vi "TestCloneAPI.vi"() -> ()   [LabVIEW 2014, in "AnalysisModule.lvlib"]
uses:
  AnalysisModule.lvlib
  TestInfo.ctl
  <userlib>/NIST/ModuleAdminLib/CloneRegistration/CloneRegistration.lvclass
  <userlib>/NIST/ModuleAdminLib/ModuleAdmin/ModuleAdmin.lvclass/ModuleAdmin.ctl
  <userlib>/NIST/ModuleAdminLib/ModuleAdmin/ModuleAdmin.lvclass
  PublicAPI/Arguments/Broadcasts/clDidInit.ctl
  PublicAPI/Arguments/Requests/clStopArgument.ctl
  <userlib>/NIST/ModuleAdminLib/ModuleAdmin/Accessors/Read CloneRegRef.vi
  <userlib>/NIST/ModuleAdminLib/ModuleAdmin/Accessors/Write CloneRegRef.vi
  AnalysisPlugins/AnalysisPluginBaseClass/AnalysisPluginsBase.lvclass
panel:
  in  "btnPref":bool
  out "error out":errorcluster
  in  "TimeStamp":dbl format="%.6f"
  in  "btnLoadPlugin":bool
  in  "SampleDataArray":cluster{"dSampleData":dbl[], "iActualPts":i32}[](array[cluster])=[{"dSampleData"=array[4800 elements], "iActualPts"=4800}, {"dSampleData"=array[4800 elements], "iActualPts"=4800}, {"dSampleData"=array[4800 elements], "iActualPts"=4800}, {"dSampleData"=array[4800 elements], "iActualPts"=4800}, {"dSampleData"=array[4800 elements], "iActualPts"=4800}, {"dSampleData"=array[4800 elements], "iActualPts"=4800}, {"dSampleData"=array[4800 elements], "iActualPts"=4800}, {"dSampleData"=array[4800 elements], "iActualPts"=4800}]
  in  "Show Panel":bool=TRUE
  in  "Plugin Type":u16(ring) items=["None", "PMU"]
  in  "btnWriteSamples":bool
  out "Path":path
  in  "btnRequestINIPath":bool
  in  "btnRemove":bool
  out "Status Log":string
  out "Active Modules (Array)":string[](array[string])
  in  "btnAdd":bool
  in  "btnStop":bool
  in  "Select Module":i32(ring)=-1 caption="Select Module to send Request" items=["All"=-1, "4140005"=4140005]
  # "Hidden"
  # "Visible"
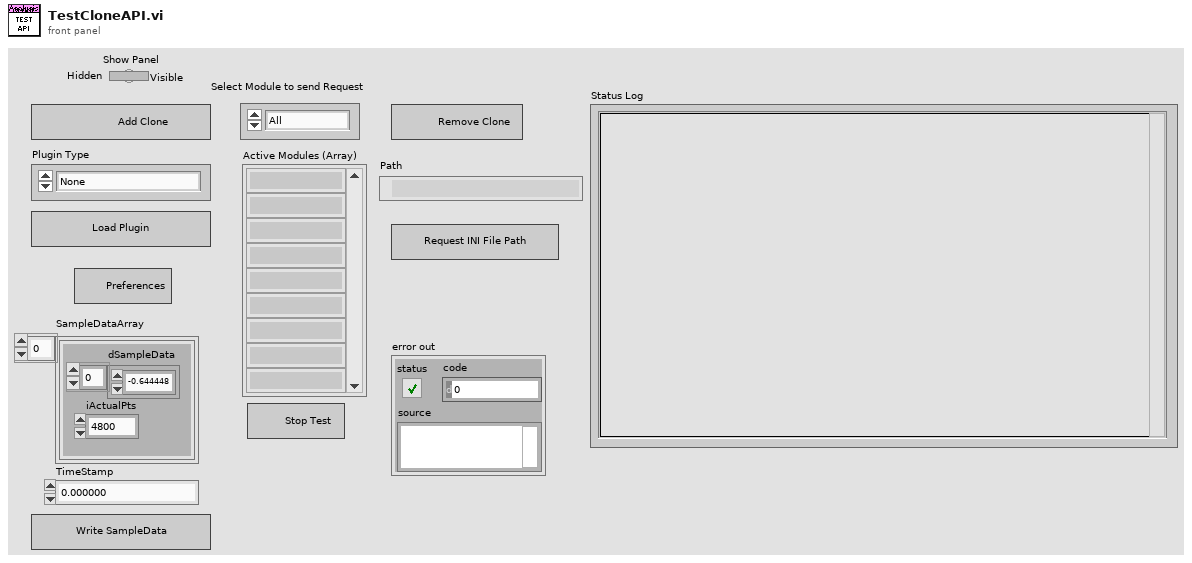
[diagram p1: front panel]
types:
  T1 = typedef "AnalysisModule.lvlib/TestInfo.ctl" = cluster{"PluginIniFilePaths":path[]}
  T2 = typedef "AnalysisModule.lvlib/clBroadcastEvents.ctl" = cluster{"DidInit":refnum<user-event>, "StatusUpdate":refnum<user-event>, "ErrorReport":refnum<user-event>, "DidStop":refnum<user-event>, "PathToINI":refnum<user-event>, "Config":refnum<user-event>, "ResultReport":refnum<user-event>}
  T3 = typedef "AnalysisModule.lvlib/clDidInit.ctl" = cluster{"Init?":bool, "ModuleAdmin":refnum<class "ModuleAdmin.lvclass">}
  T4 = typedef "AnalysisModule.lvlib/clStopArgument.ctl" = cluster{"Exit via Stop Module Req?":bool, "Wait for Module to stop?":bool, "ModuleAdmin":refnum<class "ModuleAdmin.lvclass">}
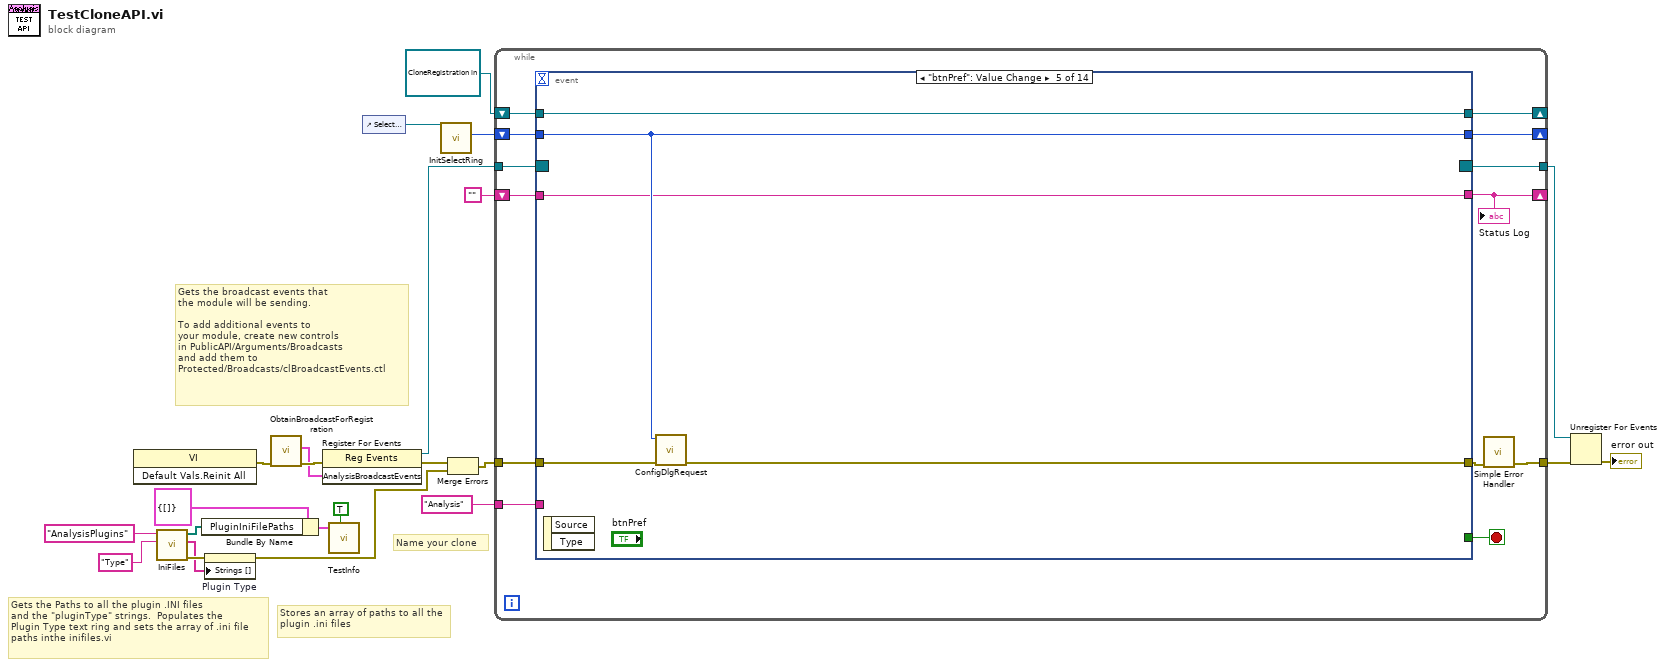
[diagram p0: block diagram]
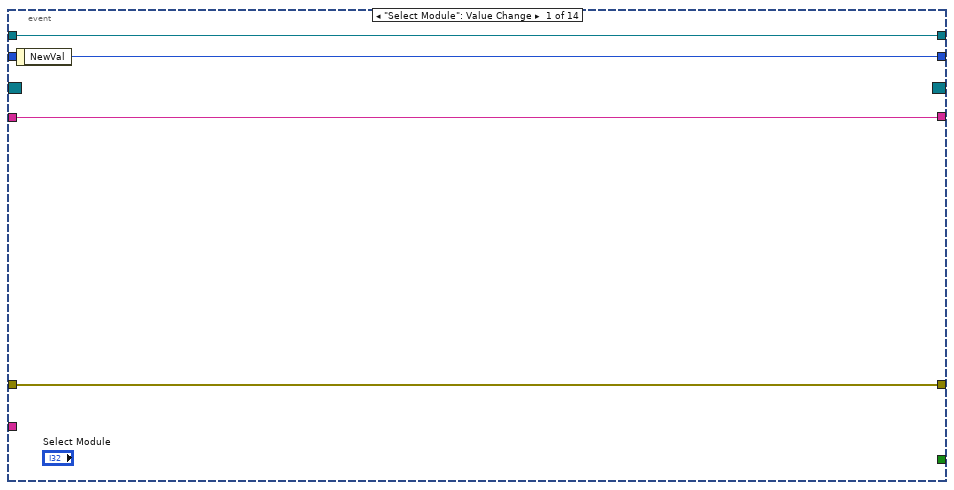
[diagram p2: hidden frame]
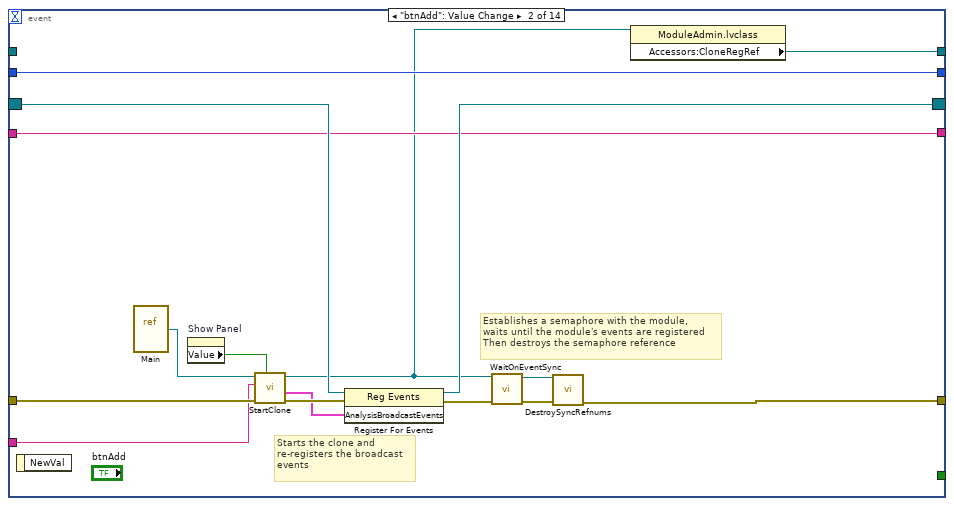
[diagram p3: hidden frame]
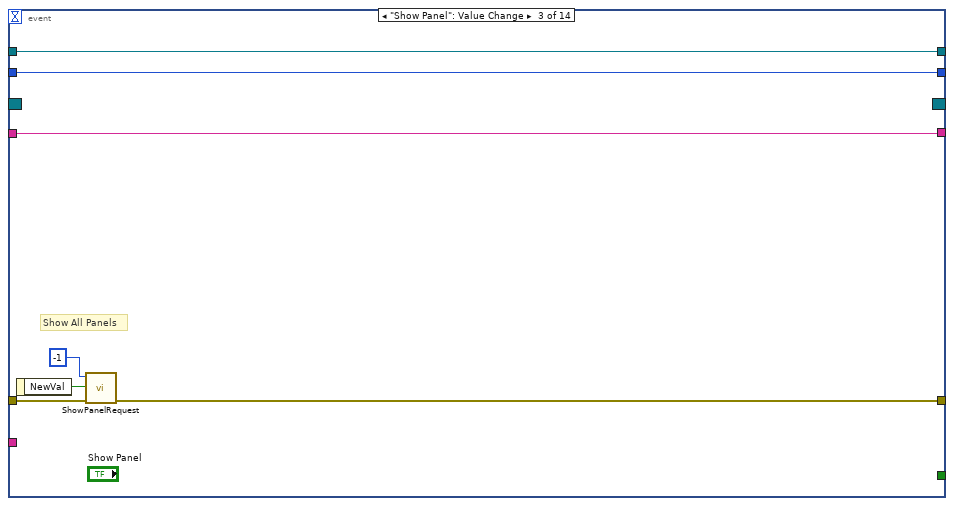
[diagram p4: hidden frame]
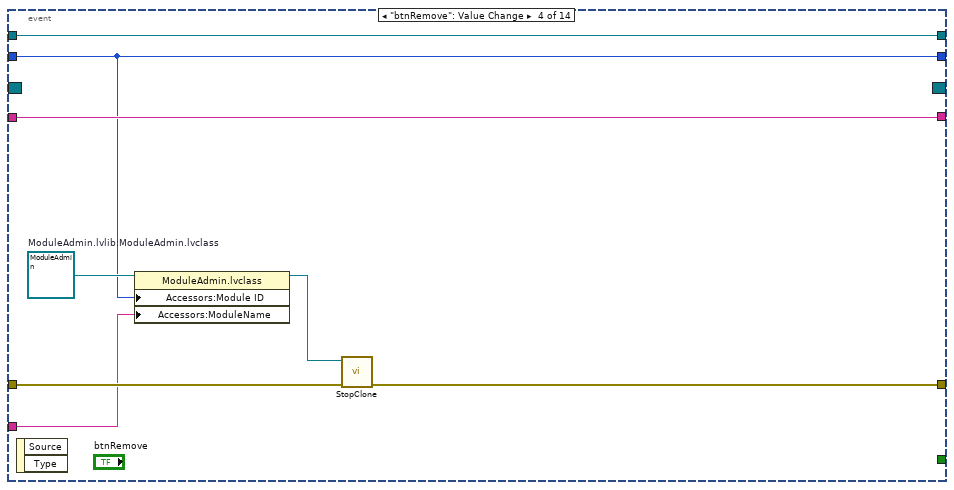
[diagram p5: hidden frame]
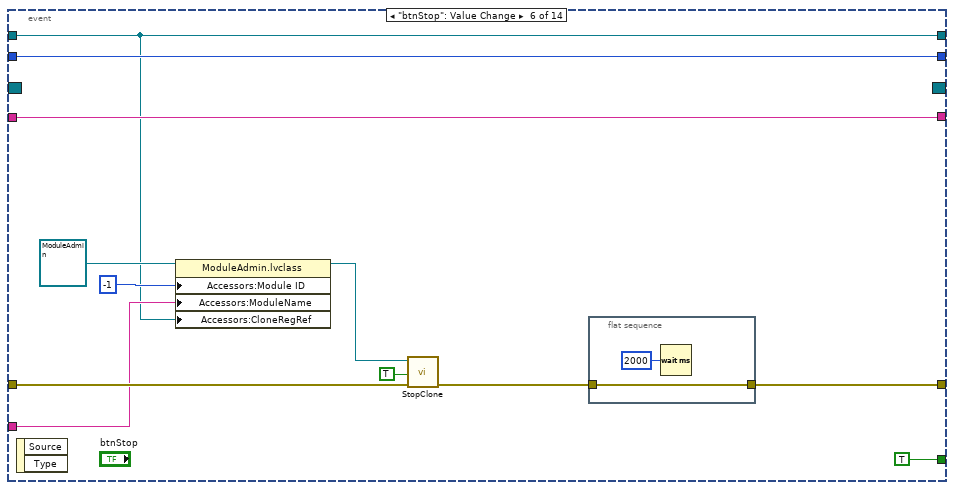
[diagram p6: hidden frame]
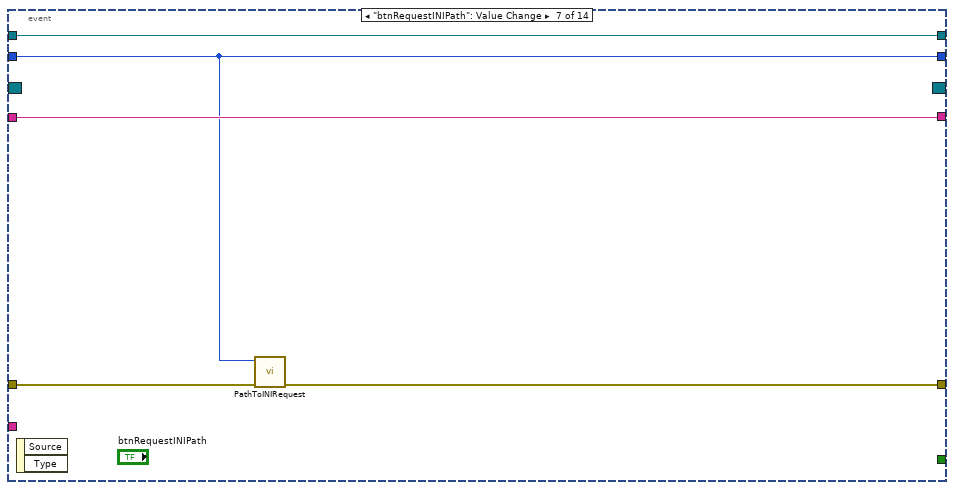
[diagram p7: hidden frame]
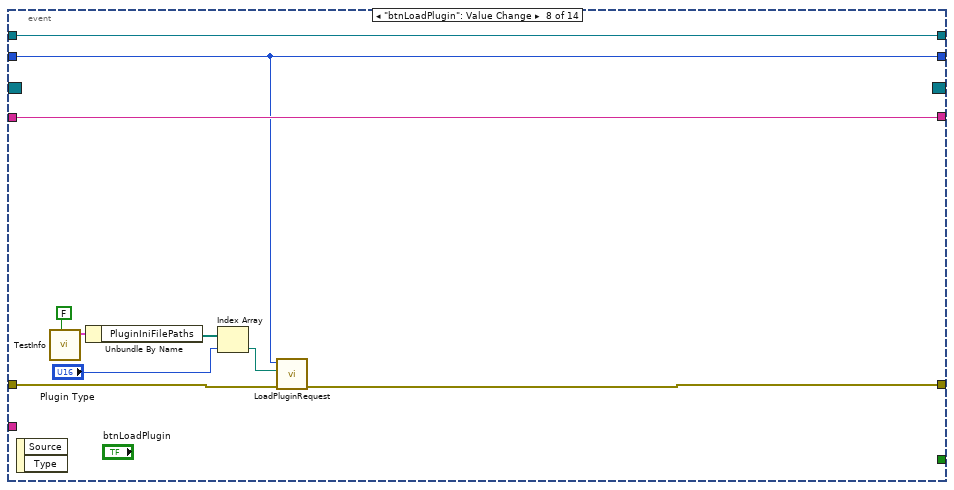
[diagram p8: hidden frame]
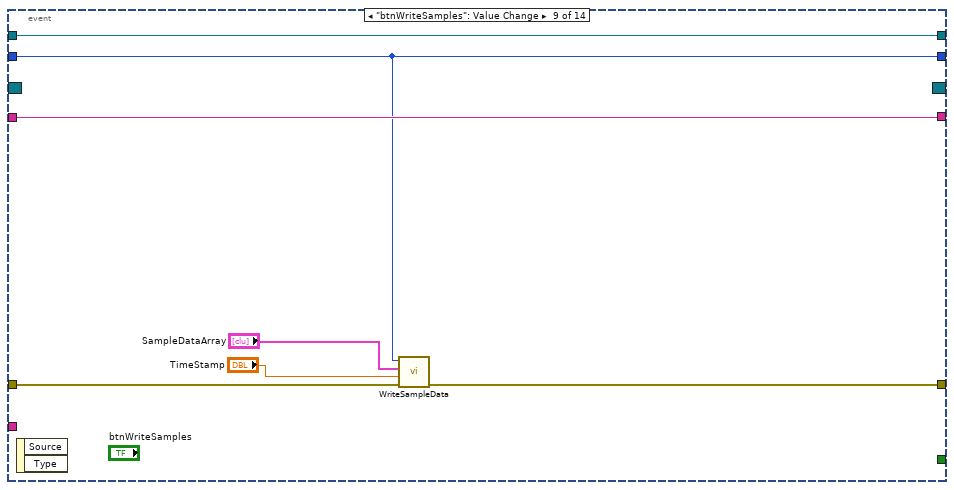
[diagram p9: hidden frame]
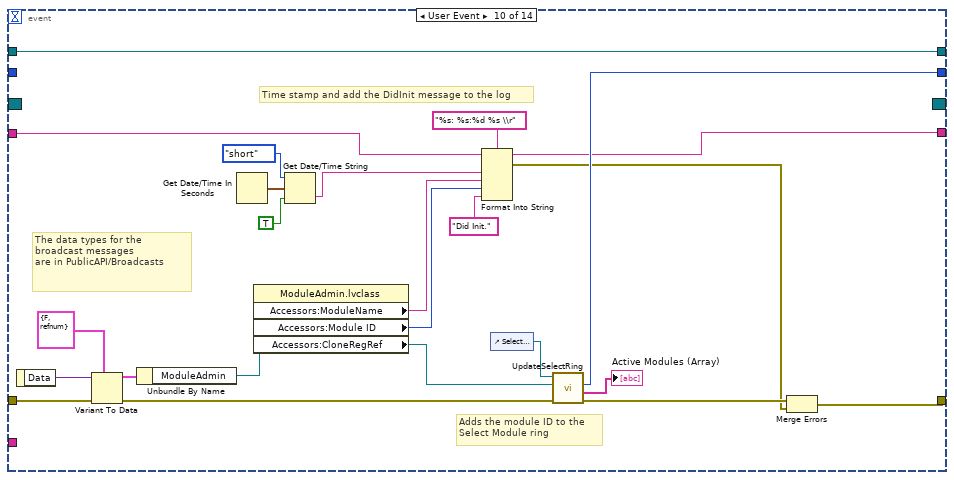
[diagram p10: hidden frame]
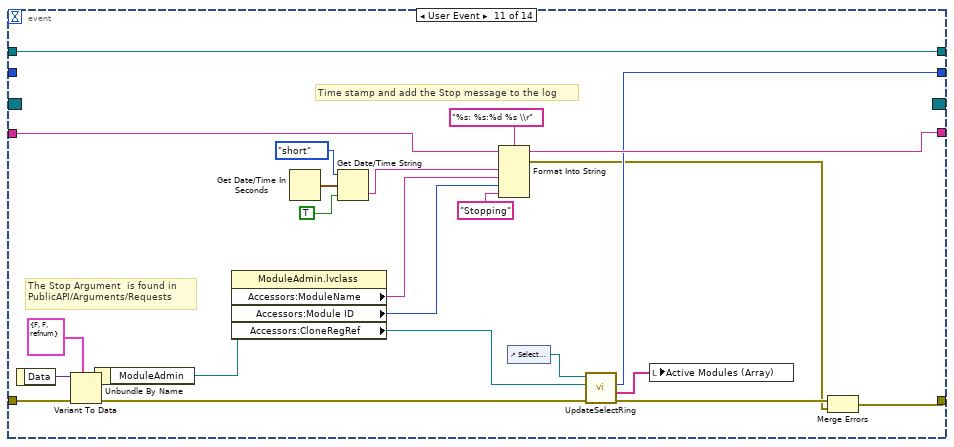
[diagram p11: hidden frame]
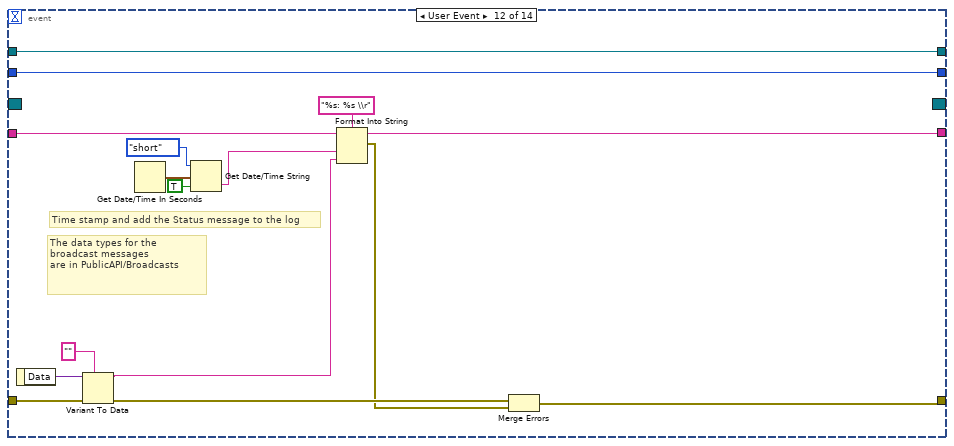
[diagram p12: hidden frame]
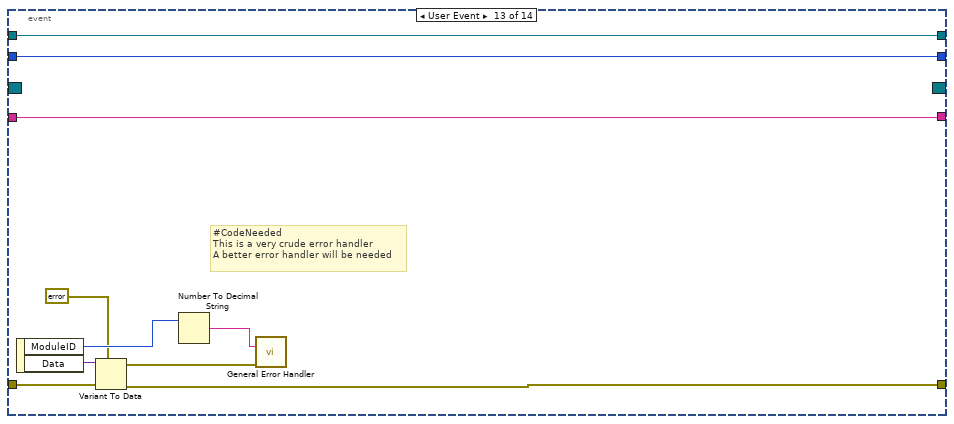
[diagram p13: hidden frame]
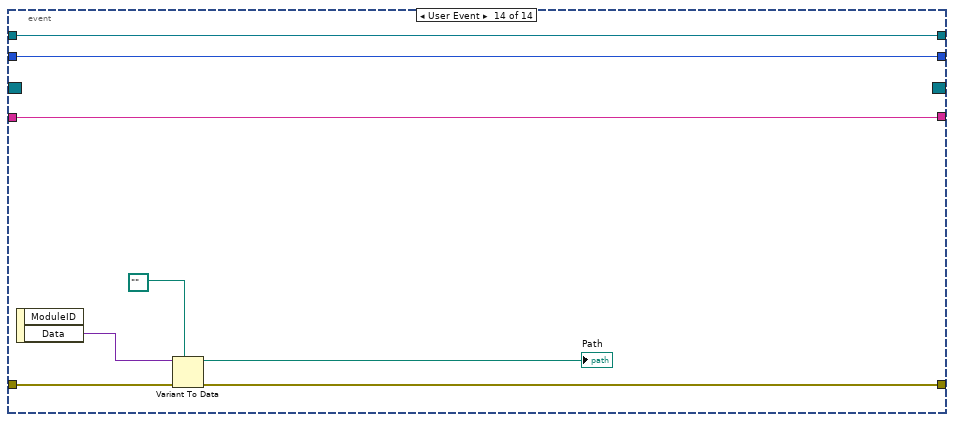
[diagram p14: hidden frame]
diagram:
  # "Stores an array of paths to all the plugin .ini files"
  # "Gets the Paths to all the plugin .INI files\nand the \"pluginType\" strings.  Populates the \nPlugin Type text ring and sets the array of .ini file\npaths inthe inifiles.vi"
  # "Name your clone"
  # "Gets the broadcast events that\nthe module will be sending.\n\nTo add additional events to\nyour module, create new controls\nin PublicAPI/Arguments/Broadcasts\nand add them to\nProtected/Broadcasts/clBroadcastEvents.ctl"
  n1 = invoke class="VI" method="Default Vals.Reinit All"() -> (error out=w21:errorcluster)  [unwired: 3 in, 2 out]
  n2 = call "IniFiles.vi"("iniKey"="Type", "name or relative path"="AnalysisPlugins") -> ("error out"=w14:errorcluster, "Types"=w13:string[], "IniFilePaths"=w12:path[])  [unwired: 7 in]
  n3 = Bundle By Name(cluster=T1 {"PluginIniFilePaths"=[]} ("TestInfo"), "PluginIniFilePaths"=w12) -> (w11:T1)
  n4 = property on="Plugin Type" class="Ring (strict)"(error in=w14, "Strings []"=w13) -> (error out=w8:errorcluster)  [unwired: 1 in, 1 out]
  n5 = call "ObtainBroadcastForRegistration.vi"("error in (no error)"=w21) -> ("error out"=w20:errorcluster, "AnalysisBroadcastEvents"=w19:T2)  [unwired: 9 in]
  n6 = register-events(error in=w20, w19) -> (reference out=w17:refnum<event-registration>, error out=w18:errorcluster)  [unwired: 1 in]
  n7 = call "TestInfo.vi"("Set (f)"=TRUE, "TestInfo 2"=w11) -> ()  [unwired: 9 in, 1 out]
  n8 = control-ref of="Select Module"() -> (w23:refnum<vi>)
  n9 = call "InitSelectRing.vi"("Ring Refnum"=w23) -> ("Module Ring Value"=w22:i32)  [unwired: 9 in, 1 out]
  n10 = Merge Errors(w18, w8) -> (w9:errorcluster)
  n11 = while {
    shift-right: [w35] -> _
    shift-left: w22 -> [w36]
    tunnel: w9 -> [w33]
    tunnel: w17 -> [w30]
    tunnel: [w31] -> w4
    shift-right: [w29] -> _
    shift-left: "" -> [w28]
    tunnel: "Analysis" ("ModuleName") -> [w27]
    tunnel: [w26] -> w3
    shift-right: [w25] -> _
    shift-left: refnum<data-value> refnum ("Accessors:CloneRegRef") -> [w24]
    stop <- w34 stop-if-true
    n12 = event shown="[4] \"btnPref\": Value Change" {
      selector: w30 -> [_ w49 _ _ _ _ _ _ _ _ _ _ _ _]
      dyn-events: [_ w48 _ _ _ _ _ _ _ _ _ _ _ _] -> w26
      timeout: _ -> [_ _ _ _ _ _ _ _ _ _ _ _ _ _]
      tunnel: w36 -> [_ w56 w59 w67 w74 w88 w94 w102 w110 _ _ w176 w181 w193]
      tunnel: [w40 w56 w59 w67 w74 w88 w94 w102 w110 w131 w147 w176 w181 w193] -> w35
      tunnel: [_ _ _ _ _ TRUE _ _ _ _ _ _ _ _] -> w34
      tunnel: w33 -> [w38 w55 w62 w70 w76 w86 w93 w104 w112 w136 w156 w173 w185 w189]
      tunnel: [w38 w43 w60 w69 w72 w79 w92 w103 w107 w120 w144 w167 w184 w188] -> w32
      tunnel: [w39 w46 w58 w71 w73 w84 w95 w105 w111 w124 w153 w170 w180 w194] -> w29
      tunnel: w28 -> [w39 w46 w58 w71 w73 w84 w95 w105 w111 w123 w154 w175 w180 w194]
      tunnel: w27 -> [_ w45 _ w66 _ w81 _ _ _ _ _ _ _ _]
      tunnel: [w37 w41 w57 w64 w75 w77 w91 w96 w106 w113 w137 w161 w177 w187] -> w25
      tunnel: w24 -> [w37 _ w57 w64 w75 w77 w91 w96 w106 w113 w137 w161 w177 w187]
      event "Select Module": Value Change {
        n13 = event-data() -> ("NewVal"=w40:i32)  [unwired: 1 in]
      }
      event "btnAdd": Value Change {
        # "Establishes a semaphore with the module,\nwaits until the module's events are registered\nThen destroys the semaphore reference"
        # "Starts the clone and\nre-registers the broadcast \nevents"
        n14 = event-data() -> ()  [unwired: 1 in, 1 out]
        n15 = vi-ref "Main.vi"() -> (w47:refnum<vi>)
        n16 = property on="Show Panel" class="Bool (strict)"() -> ("Value"=w44:bool)  [unwired: 2 in, 2 out]
        n17 = call "StartClone.vi"("ShowPanel? (f)"=w44, "error in (no error)"=w55, "ModuleName"=w45, "VI Refnum"=w47) -> ("error out"=w54:errorcluster, "AnalysisBroadcastEvents"=w50:T2, "ModuleAdmin"=w42:refnum<class "ModuleAdmin.lvclass">)  [unwired: 5 in]
        n18 = register-events(reference=w49, error in=w54, w50) -> (reference out=w48:refnum<event-registration>, error out=w53:errorcluster)
        n19 = call <userlib>:"WaitOnEventSync.vi"("error in (no error)"=w53, "ModuleAdmin"=w42) -> ("error out"=w52:errorcluster, "ModuleAdmin"=w51:refnum<class "ModuleAdmin.lvclass">)  [unwired: 8 in]
        n20 = call <userlib>:"DestroySyncRefnums.vi"("error in (no error)"=w52, "ModuleAdmin"=w51) -> ("error out"=w43:errorcluster)  [unwired: 9 in]
        n21 = property class="ModuleAdmin.lvclass"(reference=w42) -> ("Accessors:CloneRegRef"=w41:refnum<data-value>)  [unwired: 1 in, 2 out]
      }
      event "Show Panel": Value Change {
        # "Show All Panels"
        n22 = event-data() -> ("NewVal"=w63:bool)  [unwired: 1 in]
        n23 = call "ShowPanelRequest.vi"("error in (no error)"=w62, "ShowPanel?"=w63, "ModuleID"=-1) -> ("error out"=w60:errorcluster)  [unwired: 8 in]
      }
      event "btnRemove": Value Change {
        w68 = refnum<class "ModuleAdmin.lvclass"> refnum  # ModuleAdmin.lvlib:ModuleAdmin.lvclass
        n24 = event-data() -> ()  [unwired: 1 in, 2 out]
        n25 = property class="ModuleAdmin.lvclass"(reference=w68, "Accessors:Module ID"=w67, "Accessors:ModuleName"=w66) -> (reference out=w65:refnum<class "ModuleAdmin.lvclass">)  [unwired: 1 in, 1 out]
        n26 = call "StopClone.vi"("error in (no error)"=w70, "ModuleAdmin"=w65) -> ("error out"=w69:errorcluster)  [unwired: 9 in]
      }
      event "btnPref": Value Change {
        n27 = event-data() -> ()  [unwired: 1 in, 2 out]
        n28 = call "ConfigDlgRequest.vi"("error in (no error)"=w76, "ModuleID"=w74) -> ("error out"=w72:errorcluster)  [unwired: 9 in]
      }
      event "btnStop": Value Change {
        n29 = event-data() -> ()  [unwired: 1 in, 2 out]
        n30 = property class="ModuleAdmin.lvclass"(reference=refnum<class "ModuleAdmin.lvclass"> refnum ("ModuleAdmin.lvlib:ModuleAdmin.lvclass"), "Accessors:Module ID"=-1 ("Module ID"), "Accessors:ModuleName"=w81, "Accessors:CloneRegRef"=w77) -> (reference out=w80:refnum<class "ModuleAdmin.lvclass">)  [unwired: 1 in, 1 out]
        n31 = call "StopClone.vi"("error in (no error)"=w86, "Wait for Module to stop?"=TRUE, "ModuleAdmin"=w80) -> ("error out"=w78:errorcluster)  [unwired: 8 in]
        n32 = flat-sequence {
          tunnel: [w89] -> w79
          tunnel: w78 -> [w89]
          frame #0 {
            n33 = Wait (ms)(milliseconds to wait=u32 2000) -> ()  [unwired: 1 out]
          }
        }
      }
      event "btnRequestINIPath": Value Change {
        n34 = event-data() -> ()  [unwired: 1 in, 2 out]
        n35 = call "PathToINIRequest.vi"("error in (no error)"=w93, "ModuleID"=w94) -> ("error out"=w92:errorcluster)  [unwired: 9 in]
      }
      event "btnLoadPlugin": Value Change {
        n36 = event-data() -> ()  [unwired: 1 in, 2 out]
        n37 = call "TestInfo.vi"("Set (f)"=FALSE) -> ("TestInfo"=w100:T1)  [unwired: 10 in]
        n38 = Unbundle By Name(w100) -> ("PluginIniFilePaths"=w99:path[])
        n39 = Index Array(array=w99, index="Plugin Type") -> (element=w97:path)
        n40 = call "LoadPluginRequest.vi"("error in (no error)"=w104, "PathToPluginINI"=w97, "ModuleID"=w102) -> ("error out"=w103:errorcluster)  [unwired: 8 in]
      }
      event "btnWriteSamples": Value Change {
        n41 = event-data() -> ()  [unwired: 1 in, 2 out]
        n42 = call "WriteSampleData.vi"("error in (no error)"=w112, "Timestamp"="TimeStamp", "SampleDataInput"="SampleDataArray", "ModuleID"=w110) -> ("error out"=w107:errorcluster)  [unwired: 7 in]
      }
      event User Event {
        # "Adds the module ID to the \nSelect Module ring"
        # "Time stamp and add the DidInit message to the log"
        # "The data types for the broadcast messages\nare in PublicAPI/Broadcasts"
        n43 = event-data() -> ("Data"=w135:variant)  [unwired: 1 in]
        n44 = Variant To Data(error in=w136, type=T3 {"Init?"=FALSE, "ModuleAdmin"=refnum} ("clDidInit"), Variant=w135) -> (data=w128:T3, error out=w133:errorcluster)
        n45 = Unbundle By Name(w128) -> ("ModuleAdmin"=w118:refnum<class "ModuleAdmin.lvclass">)
        n46 = Get Date/Time In Seconds() -> (seconds since 1Jan1904=w126:timestamp)
        n47 = property class="ModuleAdmin.lvclass"(reference=w118) -> ("Accessors:ModuleName"=w116:string, "Accessors:Module ID"=w115:i32, "Accessors:CloneRegRef"=w114:refnum<data-value>)  [unwired: 1 in, 2 out]
        n48 = Get Date/Time String(date format (0)=enum16{"short", "long", "abbreviated"}."short", seconds (now)=w126, want seconds? (F)=TRUE) -> (time string=w129:string)  [unwired: 1 out]
        n49 = Format Into String(format string="%s: %s:%d %s \\r", initial string=w123, w129, w116, w115, "Did Init.") -> (resulting string=w124:string, error out=w121:errorcluster)  [unwired: 1 in]
        n50 = control-ref of="Select Module"() -> (w132:refnum<vi>)
        n51 = call "UpdateSelectRing.vi"("error in (no error)"=w133, "CloneRegRef"=w114, "Ring Refnum"=w132) -> ("error out"=w122:errorcluster, "ActiveModules"=→"Active Modules (Array)":string[], "Module Ring Value"=w131:i32)  [unwired: 6 in]
        n52 = Merge Errors(w122, w121) -> (w120:errorcluster)
      }
      event User Event {
        # "Time stamp and add the Stop message to the log"
        # "The Stop Argument  is found in\nPublicAPI/Arguments/Requests"
        n53 = event-data() -> ("Data"=w155:variant)  [unwired: 1 in]
        n54 = Variant To Data(error in=w156, type=T4 {"Exit via Stop Module Req?"=FALSE, "Wait for Module to stop?"=FALSE, "ModuleAdmin"=refnum} ("Stop Argument"), Variant=w155) -> (data=w151:T4, error out=w150:errorcluster)
        n55 = Unbundle By Name(w151) -> ("ModuleAdmin"=w142:refnum<class "ModuleAdmin.lvclass">)
        n56 = property class="ModuleAdmin.lvclass"(reference=w142) -> ("Accessors:ModuleName"=w140:string, "Accessors:Module ID"=w139:i32, "Accessors:CloneRegRef"=w138:refnum<data-value>)  [unwired: 1 in, 2 out]
        n57 = Get Date/Time In Seconds() -> (seconds since 1Jan1904=w158:timestamp)
        n58 = Get Date/Time String(date format (0)=enum16{"short", "long", "abbreviated"}."short", seconds (now)=w158, want seconds? (F)=TRUE) -> (time string=w160:string)  [unwired: 1 out]
        n59 = Format Into String(format string="%s: %s:%d %s \\r", initial string=w154, w160, w140, w139, "Stopping") -> (resulting string=w153:string, error out=w145:errorcluster)  [unwired: 1 in]
        n60 = control-ref of="Select Module"() -> (w149:refnum<vi>)
        n61 = call "UpdateSelectRing.vi"("error in (no error)"=w150, "CloneRegRef"=w138, "Ring Refnum"=w149) -> ("error out"=w146:errorcluster, "ActiveModules"=w148:string[], "Module Ring Value"=w147:i32)  [unwired: 6 in]
        n62 = local write "Active Modules (Array)"(w148) -> ()
        n63 = Merge Errors(w146, w145) -> (w144:errorcluster)
      }
      event User Event {
        # "Time stamp and add the Status message to the log"
        # "The data types for the broadcast messages\nare in PublicAPI/Broadcasts"
        n64 = event-data() -> ("Data"=w172:variant)  [unwired: 1 in]
        n65 = Variant To Data(error in=w173, type="", Variant=w172) -> (data=w162:string, error out=w169:errorcluster)
        n66 = Get Date/Time In Seconds() -> (seconds since 1Jan1904=w171:timestamp)
        n67 = Get Date/Time String(date format (0)=enum16{"short", "long", "abbreviated"}."short", seconds (now)=w171, want seconds? (F)=TRUE) -> (time string=w164:string)  [unwired: 1 out]
        n68 = Format Into String(format string="%s: %s \\r", initial string=w175, w164, w162) -> (resulting string=w170:string, error out=w168:errorcluster)  [unwired: 1 in]
        n69 = Merge Errors(w169, w168) -> (w167:errorcluster)
      }
      event User Event {
        # "#CodeNeeded\nThis is a very crude error handler\nA better error handler will be needed"
        n70 = event-data() -> ("ModuleID"=w183:i32, "Data"=w186:variant)  [unwired: 1 in]
        n71 = Variant To Data(error in=w185, type=errorcluster {"status"=FALSE, "code"=0, "source"=""} ("error constant"), Variant=w186) -> (data=w178:errorcluster, error out=w184:errorcluster)
        n72 = Number To Decimal String(number=w183) -> (decimal integer string=w182:string)  [unwired: 1 in]
        n73 = call <vilib>:"General Error Handler.vi"("[error source] (\" \")"=w182, "error in (no error)"=w178) -> ()  [unwired: 9 in, 5 out]
      }
      event User Event {
        n74 = event-data() -> ("Data"=w191:variant)  [unwired: 1 in, 1 out]
        n75 = Variant To Data(error in=w189, type=path "" ("Path"), Variant=w191) -> (data=→"Path":path, error out=w188:errorcluster)
      }
    }
    "Status Log" <- w29
    n76 = call <vilib>:"Simple Error Handler.vi"("error in (no error)"=w32) -> ("error out"=w31:errorcluster)  [unwired: 4 in, 4 out]
  }
  n77 = Unregister For Events(event registration refnum=w3, error in=w4) -> (error out=→"error out":errorcluster)
